vi "Setup.vi"(0 "SA Path in":refnum<class "SA 18GHz Path.lvclass">, 11 "error in (no error)":errorcluster) -> (4 "SA Path out":refnum<class "SA 18GHz Path.lvclass">, 15 "error out":errorcluster)   [LabVIEW 2023, in "RFFixtureCharact.RFPM.lvlib" / "SA 18GHz Path.lvclass"]
uses:
  SA 18GHz Path.lvclass
  C:/srd-semi-rfcal-software/AuxTools/STSRFFixtureCharactUtility/Source/Code Modules/Common/Base Classes/Path/Path.lvclass
  C:/srd-semi-rfcal-software/AuxTools/STSRFFixtureCharactUtility/Source/Code Modules/Fixture/Public/Base Classes/Scalar/SA Abstract Path/SA Abstract Path.lvclass
  Public/Base Classes/Scalar/SA Abstract Path/SA Abstract Path.lvclass/SA Abstract Path.ctl
  Public/Base Classes/Scalar/SA Abstract Path/Properties/Read Cal Tone Pin.vi
  Public/Base Classes/Scalar/SA Abstract Path/SA Abstract Path.lvclass
  Common/RFCalAndFixtureCharact.Common.lvlib
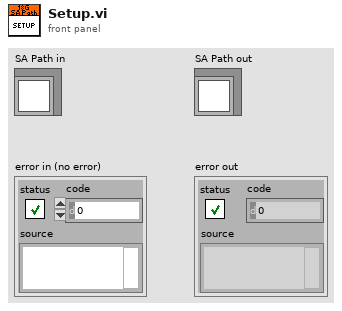
[diagram p1: front panel]
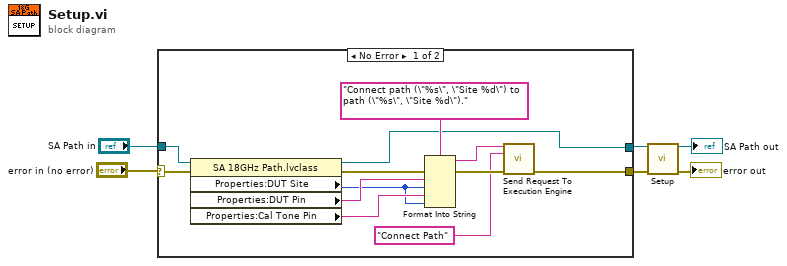
[diagram p0: block diagram]
diagram:
  n1 = case shown="No Error" "error in (no error)" {
    selector: "error in (no error)" -> [w18 w19]
    tunnel: "SA Path in" -> [w15 w20]
    tunnel: [w7 w20] -> w5
    tunnel: [w8 w19] -> w4
    frame No Error {
      n2 = property class="SA 18GHz Path.lvclass"(reference=w15, error in=w18) -> (reference out=w7:refnum<class "SA 18GHz Path.lvclass">, error out=w17:errorcluster, "Properties:DUT Site"=w13:i32, "Properties:DUT Pin"=w16:string, "Properties:Cal Tone Pin"=w14:string)
      n3 = Format Into String(format string="Connect path (\"%s\", \"Site %d\") to path (\"%s\", \"Site %d\").", error in=w17, w16, w13, w14, w13) -> (resulting string=w10:string, error out=w11:errorcluster)  [unwired: 1 in]
      n4 = call "Send Request To Execution Engine.vi"("Request Message"=w10, "Request Header"="Connect Path", "error in (no error)"=w11) -> ("error out"=w8:errorcluster)  [unwired: 11 in, 1 out]
    }
    frame Error {
    }
  }
  n5 = call-parent "Setup.vi"("Scalar SA Path in"=w5, "error in (no error)"=w4) -> ("Scalar SA Path out"=→"SA Path out":refnum<class "SA 18GHz Path.lvclass">, "error out"=→"error out":errorcluster)  [unwired: 12 in]
